vi "Trajectory Loading Polishing.vi"(6 "PID Cluster":T5={"L1 to L4 PID Cluster"={"L1 PID Gains"={"Kp"=0.005, "Kd"=0.5, "Ki"=0.0005}, "L2 PID Gains"={"Kp"=0.01, "Kd"=1.0, "Ki"=0.005}, "L3 PID Gains"={"Kp"=0.05, "Kd"=1.0, "Ki"=0.0005}, "L4 PID Gains"={"Kp"=0.1, "Kd"=0.1, "Ki"=0.0005}}, "Stage PID Cluster"={"Stage Z PID"={"Kp"=0.0005, "Kd"=0.001, "Ki"=0.0}, "Stage Y PID"={"Kp"=0.0003, "Kd"=0.01, "Ki"=0.0}, "Stage X PID"={"Kp"=0.0003, "Kd"=0.01, "Ki"=0.0}}, "OCT Z PID Gains"={"Kp"=0.0003, "Kd"=0.0001, "Ki"=0.01}}, 8 "error in":errorcluster, 9 "Offset Home 2 RCM":dbl[](array[numeric])=[0.0, 0.0, 0.0, 0.0], 10 "Prev Posit Cluster":T4={"Prev L1 to L4 Posit"=[-0.5319, -0.035669172703475985, -2.0566170657346783, 0.9099264705882353], "Prev Stage Posit"=[6.002553885707208, 5.996566124542428, 5.995469940427586], "Prev OCT Z Posit"=-0.0}, 11 "FPGA VI Reference In":refnum<k20>) -> (0 "RUY Cluster":T1, 1 "Trajectory Cluster":T2, 2 "Last Posit Cluster":T3={"Last L1 to L4 Posit"=[0.0, 0.0, 0.0, 0.0], "Last Stage Posit"=[6.0, 6.0, 6.0], "Last OCT Z Posit"=0.0}, 3 "FPGA VI Reference Out":refnum<k20>, 4 "error out":errorcluster, 5 "First Trk Pt":dbl[](array[numeric]))   [LabVIEW 2016]
uses:
  <vilib>/Platform/TimedLoop/XDataNode/timing_clust.ctl
  <vilib>/Platform/TimedLoop/XDataNode/nitl_modes.ctl
  <vilib>/Platform/TimedLoop/XDataNode/wakeup.ctl
  Global Variables.vi
  <vilib>/platform/TimedLoop/XDataNode/XDataNode.xnode
  <vilib>/Platform/TimedLoop/XDataNode/XDNodeRunTimeDep.lvlib
panel:
  out "In Servo Loop":bool
  out "Loading Finished":bool
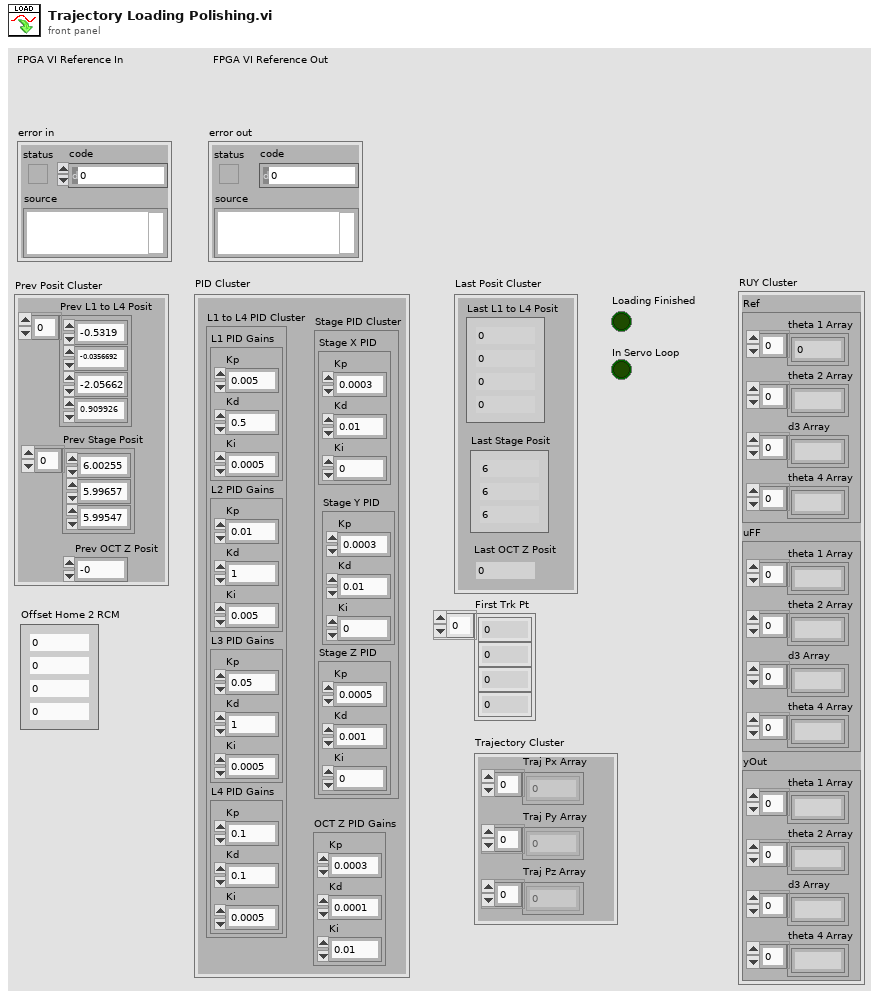
[diagram p1: front panel]
types:
  T1 = cluster{"Ref":cluster{"theta 1 Array":dbl[], "theta 2 Array":dbl[], "d3 Array":dbl[], "theta 4 Array":dbl[]}, "uFF":cluster{"theta 1 Array":dbl[], "theta 2 Array":dbl[], "d3 Array":dbl[], "theta 4 Array":dbl[]}, "yOut":cluster{"theta 1 Array":dbl[], "theta 2 Array":dbl[], "d3 Array":dbl[], "theta 4 Array":dbl[]}}
  T2 = cluster{"Traj Px Array":dbl[], "Traj Py Array":dbl[], "Traj Pz Array":dbl[]}
  T3 = cluster{"Last L1 to L4 Posit":dbl[], "Last Stage Posit":dbl[], "Last OCT Z Posit":dbl}
  T4 = cluster{"Prev L1 to L4 Posit":dbl[], "Prev Stage Posit":dbl[], "Prev OCT Z Posit":dbl}
  T5 = cluster{"L1 to L4 PID Cluster":cluster{"L1 PID Gains":cluster{"Kp":dbl, "Kd":dbl, "Ki":dbl}, "L2 PID Gains":cluster{"Kp":dbl, "Kd":dbl, "Ki":dbl}, "L3 PID Gains":cluster{"Kp":dbl, "Kd":dbl, "Ki":dbl}, "L4 PID Gains":cluster{"Kp":dbl, "Kd":dbl, "Ki":dbl}}, "Stage PID Cluster":cluster{"Stage Z PID":cluster{"Kp":dbl, "Kd":dbl, "Ki":dbl}, "Stage Y PID":cluster{"Kp":dbl, "Kd":dbl, "Ki":dbl}, "Stage X PID":cluster{"Kp":dbl, "Kd":dbl, "Ki":dbl}}, "OCT Z PID Gains":cluster{"Kp":dbl, "Kd":dbl, "Ki":dbl}}
  T6 = typedef "XDNodeRunTimeDep.lvlib/timing_clust.ctl" = cluster{"Expected End [f-1]":u64, "Actual End [f-1]":u64, "Finished Late? [f-1]":bool, "Expected End [i-1]":u64, "Actual End [i-1]":u64, "Finished Late? [i-1]":bool, "Expected Start [i]":u64, "Actual Start [i]":u64, "Expected Start [f]":u64, "Actual Start [f]":u64, "Source Name":string, "Structure Name":string, "Period":i64, "Deadline":i64, "Offset":i64, "Start":i64, "Priority":i32, "Timeout":i32, "Mode":T7, "Wakeup Reason":T8, "Error":errorcluster, "Source Type":string, "Secondary Source Type":string, "Global End Time":u64, "Global Start Time":u64, "Frame Duration":u64, "Iteration Duration":u64, "Assigned CPU":i32, "I/O Scan Engine Mode":u32}
  T7 = typedef "XDNodeRunTimeDep.lvlib/nitl_modes.ctl" = enum32{"No Change", "Process missed periods, maintain original phase", "Discard missed periods, maintain original phase", "Process missed periods, ignore original phase", "Discard missed periods, ignore original phase"}
  T8 = typedef "XDNodeRunTimeDep.lvlib/wakeup.ctl" = enum32{"Normal", "Aborted", "Asynchronous wakeup", "Timing source error", "Timed loop error", "Timeout"}
  T9 = cluster{"theta 1 Array":dbl[], "theta 2 Array":dbl[], "d3 Array":dbl[], "theta 4 Array":dbl[]}
  T10 = cluster{"L1 PID Gains":cluster{"Kp":dbl, "Kd":dbl, "Ki":dbl}, "L2 PID Gains":cluster{"Kp":dbl, "Kd":dbl, "Ki":dbl}, "L3 PID Gains":cluster{"Kp":dbl, "Kd":dbl, "Ki":dbl}, "L4 PID Gains":cluster{"Kp":dbl, "Kd":dbl, "Ki":dbl}}
  T11 = cluster{"Stage Z PID":cluster{"Kp":dbl, "Kd":dbl, "Ki":dbl}, "Stage Y PID":cluster{"Kp":dbl, "Kd":dbl, "Ki":dbl}, "Stage X PID":cluster{"Kp":dbl, "Kd":dbl, "Ki":dbl}}
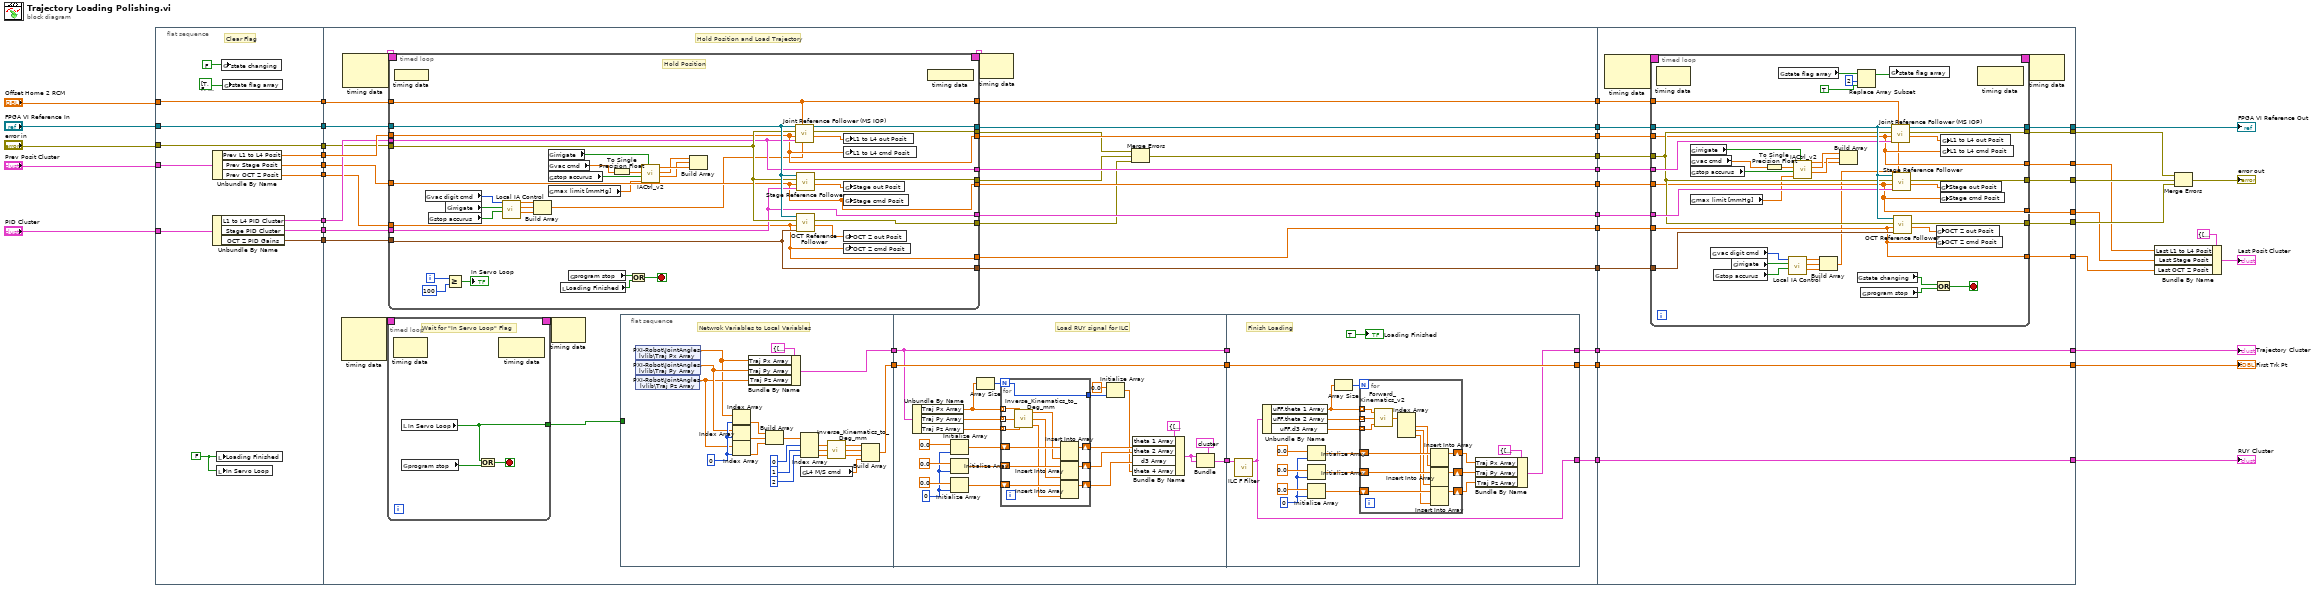
[diagram p0: block diagram]
diagram:
  n1 = flat-sequence {
    tunnel: [w51] -> w39
    tunnel: "FPGA VI Reference In" -> [w51]
    tunnel: [w50] -> w37
    tunnel: "error in" -> [w50]
    tunnel: "Prev Posit Cluster" -> [w49]
    tunnel: "PID Cluster" -> [w48]
    tunnel: [w47] -> w35
    tunnel: [w46] -> w34
    tunnel: "Offset Home 2 RCM" -> [w45]
    tunnel: [w45] -> w32
    tunnel: [w44] -> w29
    tunnel: [w43] -> w28
    tunnel: [w42] -> w27
    tunnel: [w41] -> w26
    tunnel: w39 -> [w73]
    tunnel: w37 -> [w68]
    tunnel: w35 -> [w70]
    tunnel: w34 -> [w69]
    tunnel: w32 -> [w74]
    tunnel: w29 -> [w72]
    tunnel: w28 -> [w67]
    tunnel: w27 -> [w66]
    tunnel: w26 -> [w71]
    tunnel: [w87] -> w14
    tunnel: [w86] -> w13
    tunnel: [w85] -> w12
    tunnel: [w84] -> w11
    tunnel: [w83] -> w10
    tunnel: [w82] -> w9
    tunnel: [w81] -> w8
    tunnel: [w80] -> w7
    tunnel: [w62] -> w6
    tunnel: [w61] -> w5
    tunnel: [w60] -> w4
    tunnel: [w54] -> w2
    tunnel: w14 -> [w244]
    tunnel: [w243] -> w24
    tunnel: [w242] -> w23
    tunnel: [w241] -> w22
    tunnel: w13 -> [w240]
    tunnel: w12 -> [w239]
    tunnel: w11 -> [w238]
    tunnel: w10 -> [w237]
    tunnel: w9 -> [w236]
    tunnel: w8 -> [w235]
    tunnel: w7 -> [w234]
    tunnel: [w233] -> w20
    tunnel: [w232] -> w19
    tunnel: [w231] -> w18
    tunnel: [w230] -> w16
    tunnel: [w227] -> w15
    tunnel: w6 -> [w229]
    tunnel: w5 -> [w227]
    tunnel: [w228] -> w3
    tunnel: w4 -> [w228]
    tunnel: w2 -> [w226]
    tunnel: [w226] -> w1
    frame #0 {
      w40 = FALSE ("Loading Finished")
      # "Clear Flag"
      n2 = Unbundle By Name(w48) -> ("L1 to L4 PID Cluster"=w46:T10, "Stage PID Cluster"=w47:T11, "OCT Z PID Gains"=w41:cluster{"Kp":dbl, "Kd":dbl, "Ki":dbl})
      n3 = Unbundle By Name(w49) -> ("Prev L1 to L4 Posit"=w44:dbl[], "Prev Stage Posit"=w43:dbl[], "Prev OCT Z Posit"=w42:dbl)
      n4 = local write "Loading Finished"(w40) -> ()
      n5 = local write "In Servo Loop"(w40) -> ()
      n6 = global write "Global Variables.vi" "state changing"(FALSE ("state changing")) -> ()
      n7 = global write "Global Variables.vi" "state flag array"(bool[] [TRUE, FALSE, FALSE, FALSE, FALSE, FALSE, FALSE, FALSE, FALSE] ("state flag array")) -> ()
    }
    frame #1 {
      # "Hold Position and Load Trajectory"
      n8 = node-c288() -> (w77:T6)  [unwired: 3 in]
      n9 = node-c288() -> (w79:T6)  [unwired: 2 in]
      n10 = timed-loop {
        timing: w77 -> [_]
        timing-out: [_] -> w76
        tunnel: [w89] -> w75
        stop <- w90 stop-if-true
        # "Wait for \"In Servo Loop\" Flag"
        n11 = node-c288() -> ()  [unwired: 1 in, 1 out]
        n12 = local read "In Servo Loop"() -> (w89:bool)
        n13 = global read "Global Variables.vi" "program stop"() -> (w88:bool)
        n14 = Or(x=w89, y=w88) -> (x .or. y?=w90:bool)
        n15 = node-c288() -> ()  [unwired: 1 in, 1 out]
      }
      n16 = timed-loop {
        timing: w79 -> [_]
        timing-out: [_] -> w78
        tunnel: w72 -> [w202]
        tunnel: w67 -> [w201]
        tunnel: w70 -> [w206]
        tunnel: w69 -> [w207]
        tunnel: w68 -> [w217]
        tunnel: w73 -> [w218]
        tunnel: w74 -> [w213]
        tunnel: w66 -> [w200]
        tunnel: w71 -> [w208]
        tunnel: [w202] -> w85
        tunnel: [w201] -> w84
        tunnel: [w200] -> w83
        tunnel: [w213] -> w86
        tunnel: [w212] -> w87
        tunnel: [w211] -> w65
        tunnel: [w210] -> w64
        tunnel: [w209] -> w63
        tunnel: [w208] -> w82
        tunnel: [w207] -> w81
        tunnel: [w206] -> w80
        i -> [w205]
        stop <- w221 stop-if-true
        # "Hold Position"
        n17 = node-c288 ("Output Node")() -> ()  [unwired: 1 in]
        n18 = global read "Global Variables.vi" "vac digit cmd"() -> (w190:i8)
        n19 = global read "Global Variables.vi" "stop accurus"() -> (w189:bool)
        n20 = global read "Global Variables.vi" "irrigate"() -> (w191:bool)
        n21 = Greater Or Equal?(x=w205, y=100) -> (x >= y?=→"In Servo Loop":bool)
        n22 = call "Local IA Control.vi"("E-Stop Vacuum"=w189, "Irrigate?"=w191, "8bit integer"=w190) -> ("Accurus Engaged Vout"=w186:dbl, "Accurus ChB Vout"=w187:dbl, "Accurus ChA Vout"=w188:dbl)  [unwired: 6 in]
        n23 = Build Array(w188, w187, w186) -> (w185:dbl[])
        n24 = global read "Global Variables.vi" "irrigate"() -> (w198:bool)
        n25 = global read "Global Variables.vi" "vac cmd"() -> (w193:sgl)
        n26 = global read "Global Variables.vi" "stop accurus"() -> (w195:bool)
        n27 = global read "Global Variables.vi" "max limit [mmHg]"() -> (w192:dbl)
        n28 = local read "Loading Finished"() -> (w220:bool)
        n29 = global read "Global Variables.vi" "program stop"() -> (w219:bool)
        n30 = To Single Precision Float(number=w193) -> (single precision float=w194:sgl)
        n31 = Or(x=w219, y=w220) -> (x .or. y?=w221:bool)
        n32 = call "IACtrl_v2.vi"("Irrigate?"=w198, "Max Limit [mmHg]"=w192, "E-Stop Vacuum"=w195, "Vacuum Force [mmHg]"=w194) -> ("Accurus ChB Vout"=w196:dbl, "Accurus ChA Vout"=w197:dbl, "Accurus Engaged Vout"=w199:dbl)  [unwired: 4 in, 1 out]
        n33 = Build Array(w197, w196, w199) -> ()  [unwired: 1 out]
        n34 = call "Joint Reference Follower (MS IOP).vi"("Acc Ctrl Array"=w185, "Offset Home2RCM [deg/mm]"=w213, "PID Ctrl Cluster"=w207, "Ref Array [deg/mm]"=w202, "error in"=w217, "FPGA VI Reference In"=w218) -> ("Output Posit Array [deg/mm]"=w216:dbl[], "error out"=w211:errorcluster, "FPGA VI Reference Out"=w212:refnum<k20>)  [unwired: 3 in]
        n35 = call "Stage Reference Follower.vi"("Stage PID Cluster"=w206, "Stage cmd Posit [mm]"=w201, "error in"=w217, "FPGA VI Reference In"=w218) -> ("Stage out Posit [mm]"=w215:dbl[], "error out"=w210:errorcluster)  [unwired: 5 in, 1 out]
        n36 = call "OCT Reference Follower.vi"("OCT Z PID Gains"=w208, "OCT  Z cmd Posit [mm]"=w200, "error in"=w217, "FPGA VI Reference In"=w218) -> ("OCT  Z out Posit [mm]"=w214:dbl, "error out"=w209:errorcluster)  [unwired: 5 in, 1 out]
        n37 = global write "Global Variables.vi" "OCT Z out Posit"(w214) -> ()
        n38 = global write "Global Variables.vi" "OCT Z cmd Posit"(w200) -> ()
        n39 = global write "Global Variables.vi" "L1 to L4 out Posit"(w216) -> ()
        n40 = global write "Global Variables.vi" "L1 to L4 cmd Posit"(w202) -> ()
        n41 = global write "Global Variables.vi" "Stage out Posit"(w215) -> ()
        n42 = global write "Global Variables.vi" "Stage cmd Posit"(w201) -> ()
        n43 = node-c288() -> ()  [unwired: 1 out]
      }
      n44 = node-c288(w76) -> ()  [unwired: 1 out]
      n45 = flat-sequence {
        tunnel: [w114] -> w59
        tunnel: w75 -> [_]
        tunnel: [w97] -> w57
        tunnel: w59 -> [w126]
        tunnel: [w126] -> w58
        tunnel: w57 -> [w138]
        tunnel: [w138] -> w56
        tunnel: [w120] -> w55
        tunnel: w58 -> [_]
        tunnel: [w152] -> w61
        tunnel: [w170] -> w60
        tunnel: w56 -> [w170]
        tunnel: w55 -> [w169]
        tunnel: [w168] -> w54
        frame #0 {
          w112 = 0 ("index")
          # "Netwrok Variables to Local Variables"
          n46 = shared-variable "PXI-Robot\\JointAngles.lvlib\\Traj Px Array"() -> (w95:dbl[])  [unwired: 1 in, 1 out]
          n47 = shared-variable "PXI-Robot\\JointAngles.lvlib\\Traj Py Array"() -> (w99:dbl[])  [unwired: 1 in, 1 out]
          n48 = shared-variable "PXI-Robot\\JointAngles.lvlib\\Traj Pz Array"() -> (w98:dbl[])  [unwired: 1 in, 1 out]
          n49 = Index Array(array=w95, index=w112) -> (element=w100:dbl)
          n50 = Index Array(array=w99, index=w112) -> (element=w101:dbl)
          n51 = Index Array(array=w98, index=w112) -> (element=w102:dbl)
          n52 = Bundle By Name(cluster=T2 {"Traj Px Array"=[], "Traj Py Array"=[], "Traj Pz Array"=[]} ("Trajectory Cluster"), "Traj Px Array"=w95, "Traj Py Array"=w99, "Traj Pz Array"=w98) -> (w114:T2)
          n53 = Build Array(w100, w101, w102) -> (w113:dbl[])
          n54 = global read "Global Variables.vi" "L4 M/S cmd"() -> (w96:dbl)
          n55 = Index Array(array=w113, index #1=0 ("index"), index #2=1 ("index"), index #3=2 ("index")) -> (element #1=w107:dbl, element #2=w109:dbl, element #3=w108:dbl)
          n56 = call "Inverse_Kinematics_to_Deg_mm.vi"("pz"=w108, "py"=w109, "px"=w107) -> ("L3 [mm]"=w104:dbl, "L2 [deg]"=w105:dbl, "L1 [deg]"=w106:dbl)
          n57 = Build Array(w106, w105, w104, w96) -> (w97:dbl[])
        }
        frame #1 {
          w130 = 0 ("dimension size")
          # "Load RUY signal for ILC"
          n58 = Unbundle By Name(w126) -> ("Traj Px Array"=w136:dbl[], "Traj Py Array"=w134:dbl[], "Traj Pz Array"=w135:dbl[])
          n59 = Initialize Array(0.0 ("element"), w130) -> (w129:dbl[])
          n60 = Initialize Array(0.0 ("element"), w130) -> (w128:dbl[])
          n61 = Initialize Array(0.0 ("element"), w130) -> (w127:dbl[])
          n62 = Array Size(array=w136) -> (size(s)=w137:i32)
          n63 = for {
            N: w137 -> [w139]
            tunnel: w136 -> [w151] mode=indexing
            tunnel: w135 -> [w150] mode=indexing
            tunnel: w134 -> [w149] mode=indexing
            shift-right: [w142] -> w119
            shift-left: w129 -> [w148]
            shift-right: [w141] -> w117
            shift-left: w128 -> [w146]
            shift-right: [w140] -> w118
            shift-left: w127 -> [w144]
            tunnel: [w139] -> w123
            n64 = call "Inverse_Kinematics_to_Deg_mm.vi"("pz"=w150, "py"=w149, "px"=w151) -> ("L3 [mm]"=w143:dbl, "L2 [deg]"=w145:dbl, "L1 [deg]"=w147:dbl)
            n65 = Insert Into Array(array=w148, new element=w147) -> (w142:dbl[])  [unwired: 1 in]
            n66 = Insert Into Array(array=w146, new element=w145) -> (w141:dbl[])  [unwired: 1 in]
            n67 = Insert Into Array(array=w144, new element=w143) -> (w140:dbl[])  [unwired: 1 in]
          }
          n68 = Initialize Array(0.0 ("element"), w123) -> (w116:dbl[])
          n69 = Bundle By Name(cluster=T9 {"theta 1 Array"=[], "theta 2 Array"=[], "d3 Array"=[], "theta 4 Array"=[]} ("uFF"), "theta 1 Array"=w119, "theta 2 Array"=w117, "d3 Array"=w118, "theta 4 Array"=w116) -> (w121:T9)
          n70 = Bundle(cluster=T1 {"Ref"={"theta 1 Array"=array[6000 elements], "theta 2 Array"=array[6000 elements], "d3 Array"=array[6000 elements], "theta 4 Array"=array[6000 elements]}, "uFF"={"theta 1 Array"=array[6000 elements], "theta 2 Array"=array[6000 elements], "d3 Array"=array[6000 elements], "theta 4 Array"=array[6000 elements]}, "yOut"={"theta 1 Array"=[], "theta 2 Array"=[], "d3 Array"=[], "theta 4 Array"=[]}} ("Cluster"), "Ref"=w121, "uFF"=w121) -> (w120:T1)  [unwired: 1 in]
        }
        frame #2 {
          w164 = 0 ("dimension size")
          # "Finish Loading"
          n71 = call "ILC F Filter.vi"("Input RUY Signals"=w169) -> ("Updated RUY"=w168:T1)  [unwired: 10 in]
          n72 = Unbundle By Name(w168) -> ("uFF.theta 1 Array"=w160:dbl[], "uFF.theta 2 Array"=w163:dbl[], "uFF.d3 Array"=w162:dbl[])
          n73 = Initialize Array(0.0 ("element"), w164) -> (w159:dbl[])
          n74 = Initialize Array(0.0 ("element"), w164) -> (w158:dbl[])
          n75 = Initialize Array(0.0 ("element"), w164) -> (w157:dbl[])
          n76 = Array Size(array=w160) -> (size(s)=w161:i32)
          n77 = for {
            N: w161 -> [_]
            tunnel: w160 -> [w184] mode=indexing
            tunnel: w163 -> [w183] mode=indexing
            tunnel: w162 -> [w182] mode=indexing
            shift-right: [w174] -> w155
            shift-left: w159 -> [w180]
            shift-right: [w173] -> w154
            shift-left: w158 -> [w179]
            shift-right: [w172] -> w153
            shift-left: w157 -> [w178]
            n78 = call "Forward_Kinematics_v2.vi"("theta 3"=w182, "theta 2"=w183, "theta 1"=w184) -> ("position"=w181:dbl[])
            n79 = Index Array(array=w181) -> (element #1=w177:dbl, element #2=w176:dbl, element #3=w175:dbl)  [unwired: 3 in]
            n80 = Insert Into Array(array=w180, new element=w177) -> (w174:dbl[])  [unwired: 1 in]
            n81 = Insert Into Array(array=w179, new element=w176) -> (w173:dbl[])  [unwired: 1 in]
            n82 = Insert Into Array(array=w178, new element=w175) -> (w172:dbl[])  [unwired: 1 in]
          }
          n83 = Bundle By Name(cluster=T2 {"Traj Px Array"=[], "Traj Py Array"=[], "Traj Pz Array"=[]} ("Trajectory Cluster"), "Traj Px Array"=w155, "Traj Py Array"=w154, "Traj Pz Array"=w153) -> (w152:T2)
          "Loading Finished" <- TRUE ("Loading Finished")
        }
      }
      n84 = node-c288(w78) -> ()  [unwired: 1 out]
      n85 = Merge Errors(w65, w64, w63) -> (w62:errorcluster)
    }
    frame #2 {
      n86 = node-c288() -> (w246:T6)  [unwired: 2 in]
      n87 = timed-loop {
        timing: w246 -> [_]
        timing-out: [_] -> w245
        tunnel: w244 -> [w277]
        tunnel: [w276] -> w242
        tunnel: [w275] -> w243
        tunnel: [w274] -> w241
        tunnel: w240 -> [w273]
        tunnel: w239 -> [w264]
        tunnel: w238 -> [w263]
        tunnel: w237 -> [w262]
        tunnel: w236 -> [w272]
        tunnel: w235 -> [w271]
        tunnel: w234 -> [w270]
        tunnel: [w264] -> w233
        tunnel: [w263] -> w232
        tunnel: [w262] -> w231
        tunnel: [w266] -> w230
        tunnel: w229 -> [w265]
        stop <- w284 stop-if-true
        n88 = node-c288() -> ()  [unwired: 1 in, 1 out]
        n89 = global read "Global Variables.vi" "irrigate"() -> (w256:bool)
        n90 = global read "Global Variables.vi" "vac cmd"() -> (w261:sgl)
        n91 = global read "Global Variables.vi" "stop accurus"() -> (w259:bool)
        n92 = global read "Global Variables.vi" "max limit [mmHg]"() -> (w254:dbl)
        n93 = global read "Global Variables.vi" "vac digit cmd"() -> (w252:i8)
        n94 = global read "Global Variables.vi" "stop accurus"() -> (w251:bool)
        n95 = global read "Global Variables.vi" "irrigate"() -> (w253:bool)
        n96 = To Single Precision Float(number=w261) -> (single precision float=w260:sgl)
        n97 = global read "Global Variables.vi" "state flag array"() -> (w281:bool[])
        n98 = call "Local IA Control.vi"("E-Stop Vacuum"=w251, "Irrigate?"=w253, "8bit integer"=w252) -> ("Accurus Engaged Vout"=w248:dbl, "Accurus ChB Vout"=w249:dbl, "Accurus ChA Vout"=w250:dbl)  [unwired: 6 in]
        n99 = call "IACtrl_v2.vi"("Irrigate?"=w256, "Max Limit [mmHg]"=w254, "E-Stop Vacuum"=w259, "Vacuum Force [mmHg]"=w260) -> ("Accurus ChB Vout"=w258:dbl, "Accurus ChA Vout"=w257:dbl, "Accurus Engaged Vout"=w255:dbl)  [unwired: 4 in, 1 out]
        n100 = Build Array(w250, w249, w248) -> (w247:dbl[])
        n101 = Build Array(w257, w258, w255) -> ()  [unwired: 1 out]
        n102 = global read "Global Variables.vi" "state changing"() -> (w283:bool)
        n103 = Replace Array Subset(array=w281, new element=TRUE ("new element/subarray"), index=2) -> (w280:bool[])
        n104 = global read "Global Variables.vi" "program stop"() -> (w282:bool)
        n105 = global write "Global Variables.vi" "state flag array"(w280) -> ()
        n106 = call "Joint Reference Follower (MS IOP).vi"("Acc Ctrl Array"=w247, "Offset Home2RCM [deg/mm]"=w273, "PID Ctrl Cluster"=w271, "Ref Array [deg/mm]"=w264, "error in"=w265, "FPGA VI Reference In"=w277) -> ("Output Posit Array [deg/mm]"=w269:dbl[], "error out"=w276:errorcluster, "FPGA VI Reference Out"=w266:refnum<k20>)  [unwired: 3 in]
        n107 = call "Stage Reference Follower.vi"("Stage PID Cluster"=w270, "Stage cmd Posit [mm]"=w263, "error in"=w265, "FPGA VI Reference In"=w277) -> ("Stage out Posit [mm]"=w268:dbl[], "error out"=w275:errorcluster)  [unwired: 5 in, 1 out]
        n108 = call "OCT Reference Follower.vi"("OCT Z PID Gains"=w272, "OCT  Z cmd Posit [mm]"=w262, "error in"=w265, "FPGA VI Reference In"=w277) -> ("OCT  Z out Posit [mm]"=w267:dbl, "error out"=w274:errorcluster)  [unwired: 5 in, 1 out]
        n109 = Or(x=w283, y=w282) -> (x .or. y?=w284:bool)
        n110 = global write "Global Variables.vi" "OCT Z out Posit"(w267) -> ()
        n111 = global write "Global Variables.vi" "OCT Z cmd Posit"(w262) -> ()
        n112 = global write "Global Variables.vi" "Stage out Posit"(w268) -> ()
        n113 = global write "Global Variables.vi" "Stage cmd Posit"(w263) -> ()
        n114 = global write "Global Variables.vi" "L1 to L4 out Posit"(w269) -> ()
        n115 = global write "Global Variables.vi" "L1 to L4 cmd Posit"(w264) -> ()
        n116 = node-c288() -> ()  [unwired: 1 in, 1 out]
      }
      n117 = node-c288(w245) -> ()  [unwired: 1 out]
    }
  }
  n118 = Bundle By Name(cluster=T3 {"Last L1 to L4 Posit"=[0.0, 0.0, 0.0, 0.0], "Last Stage Posit"=[6.0, 6.0, 6.0], "Last OCT Z Posit"=0.0} ("Last Posit Cluster 2"), "Last L1 to L4 Posit"=w20, "Last Stage Posit"=w19, "Last OCT Z Posit"=w18) -> (→"Last Posit Cluster":T3)
  n119 = Merge Errors(w23, w24, w22) -> (→"error out":errorcluster)
  "FPGA VI Reference Out" <- w16
  "First Trk Pt" <- w3
  "Trajectory Cluster" <- w15
  "RUY Cluster" <- w1
